vi "LabVIEWArduino1.vi"() -> ()   [LabVIEW 2020]
uses:
  <vilib>/Instr/_visa.llb/VISA Configure Serial Port (Instr).vi
panel:
  out "GO DOWN ECHO 2":string
  out "GO UP ECHO":string
  in  "GO UP":bool
  in  "GO DOWN":bool
  out "MAX SPEED ECHO":string
  out "SLOW SPEED ECHO":string
  in  "MAX SPEED":bool
  in  "SLOWEST SPEED":bool
  out "Waveform Graph":dbl[](graph)
  in  "VISA resource name":refnum<visa-resource-name>="COM3"
  in  "data bits (8)":u16=8 min=5 max=8 step=1
  in  "stop bits (10: 1 bit)":u16(ring)=10 items=["1.0"=10, "1.5"=15, "2.0"=20]
  in  "flow control (0:none)":u16(ring) items=["None", "XON/XOFF", "RTS/CTS", "XON/XOFF & RTS/CTS", "DTR/DSR", "XON/XOFF & DTR/DSR"]
  in  "parity (0:none)":enum16{"None", "Odd", "Even", "Mark", "Space"}(ring)
  out "TempArray":dbl[](array[numeric]) caption="Temperature Array"
  out "CurTemp":dbl caption="Current Temperature\n(Celsius)"
  out "concatenated string":string
  in  "stop":bool
  in  "LabVIEW Stop":bool
  out "LabVIEW Echo":string
  out "Emergency Stop Echo":string
  in  "Emergency Stop!":bool
  out "DECELLERATE ECHO":string
  in  "Decellerate":bool
  in  "Motor Control Duino":refnum<visa-resource-name>
  out "ACCELERATE VALUE CHANGE":string
  in  "Accelerate":bool
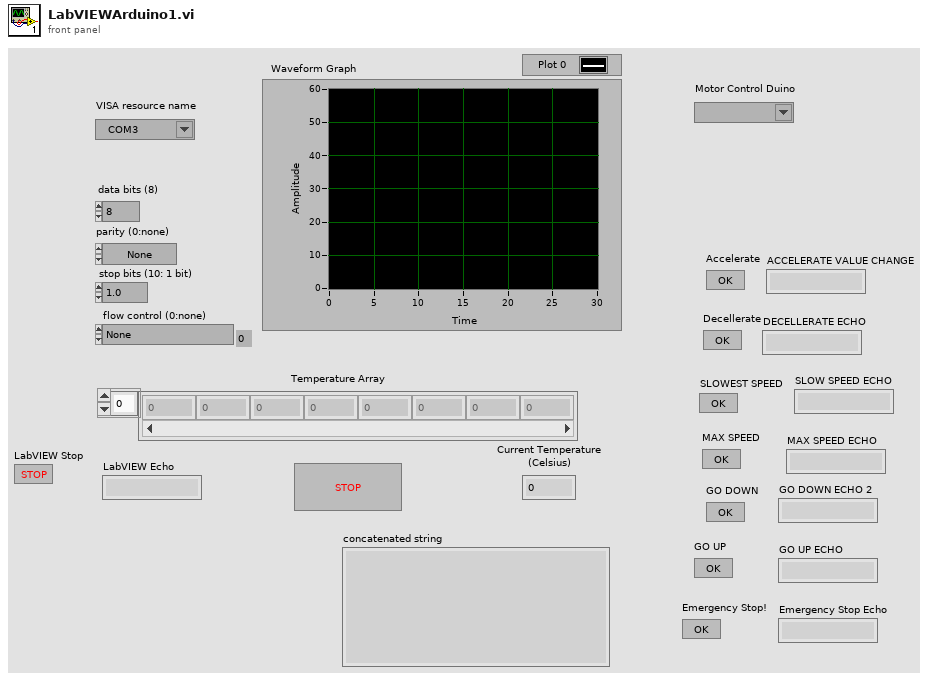
[diagram p1: front panel]
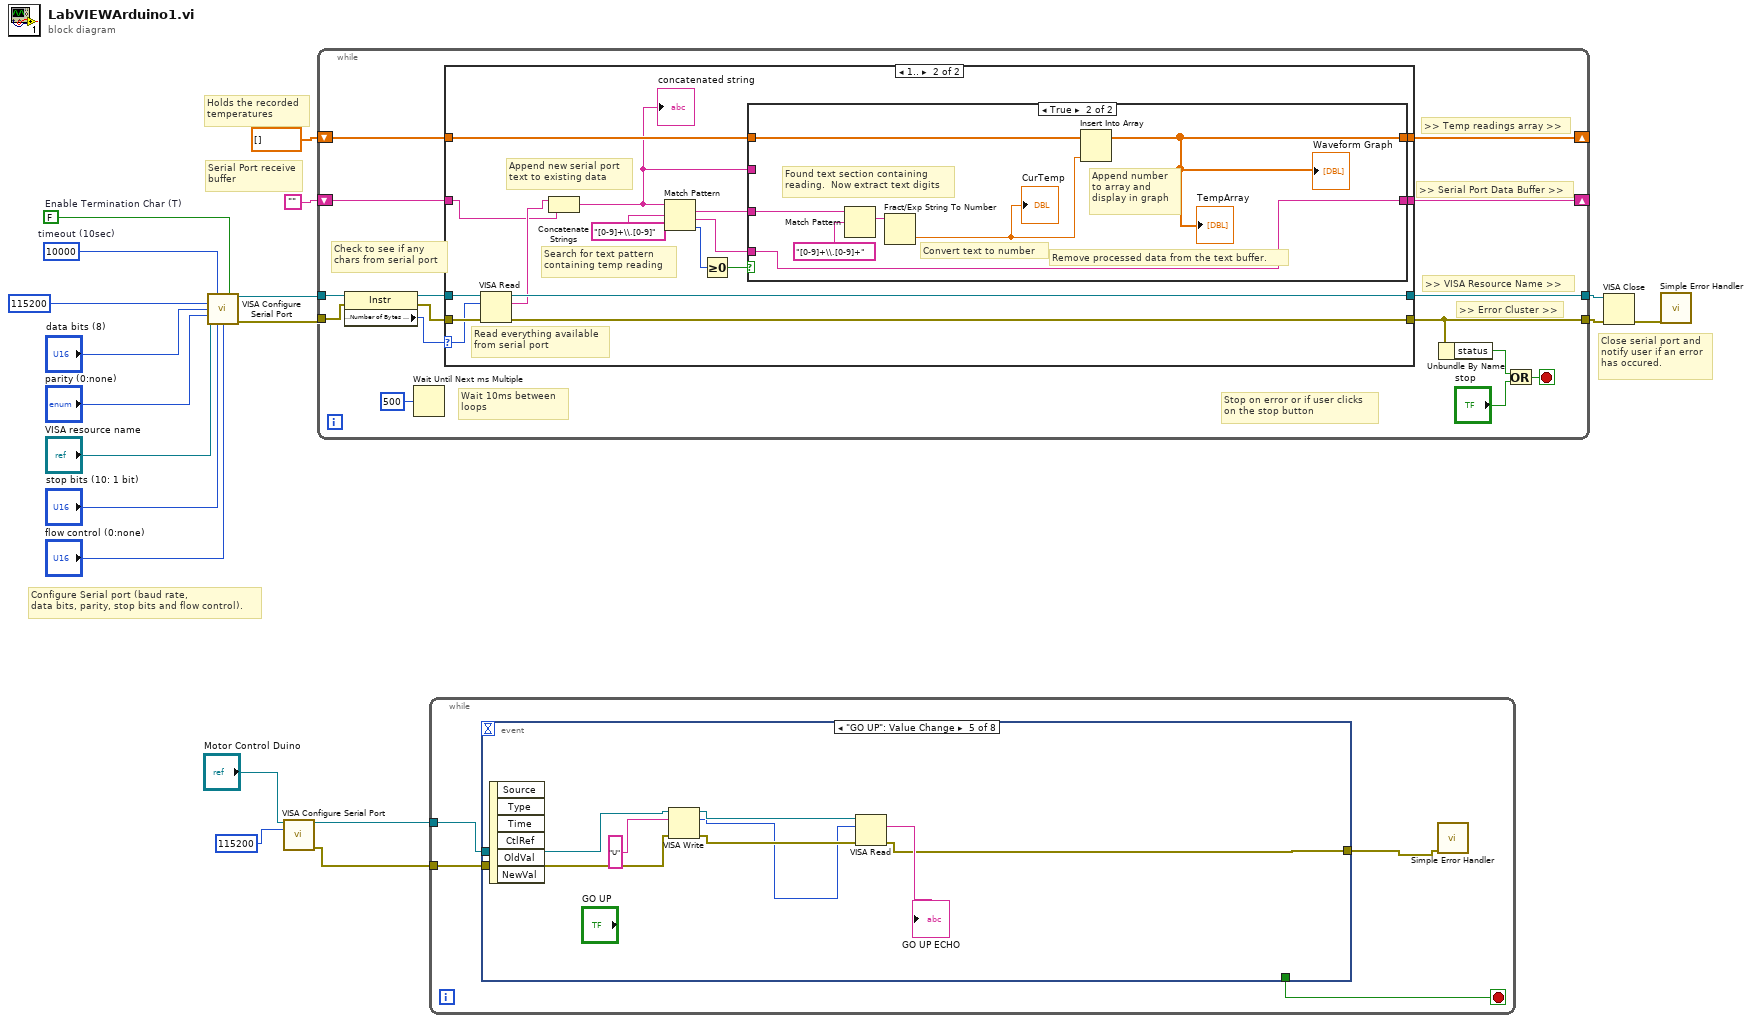
[diagram p0: block diagram]
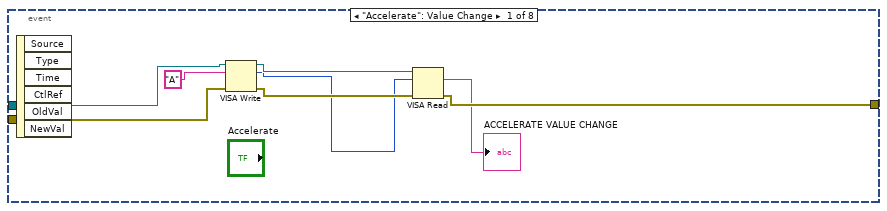
[diagram p4: hidden frame]
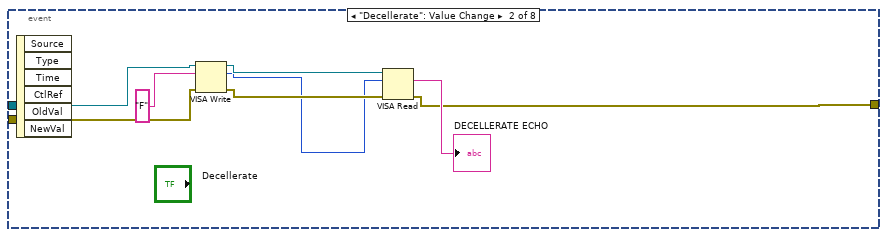
[diagram p5: hidden frame]
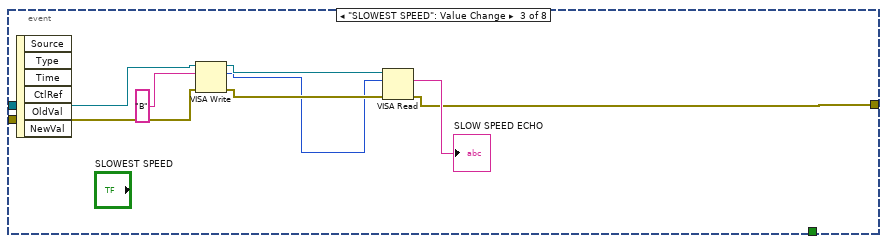
[diagram p6: hidden frame]
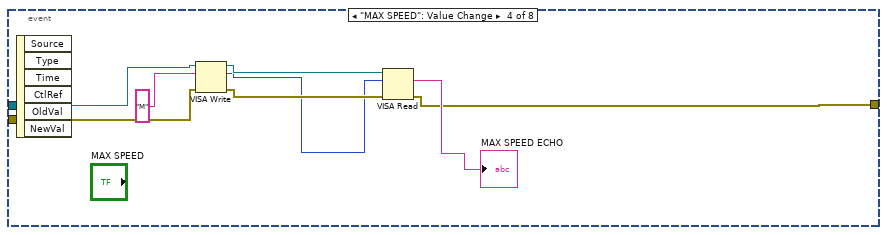
[diagram p7: hidden frame]
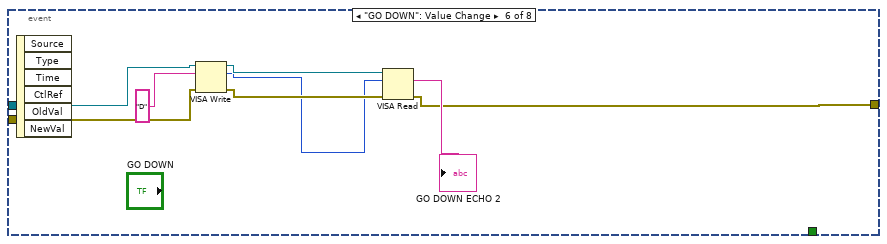
[diagram p8: hidden frame]
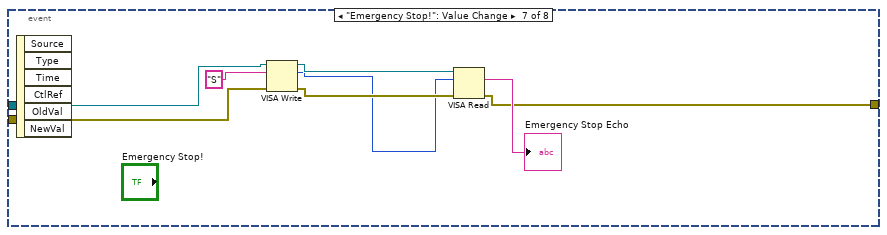
[diagram p9: hidden frame]
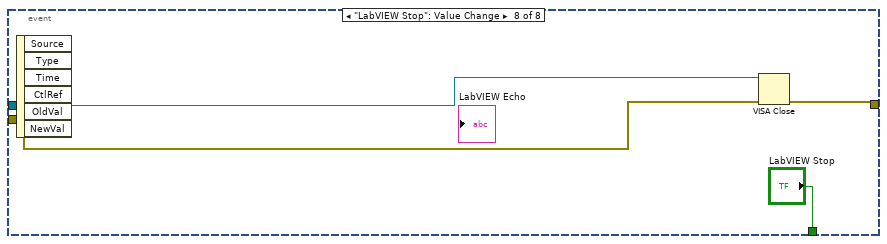
[diagram p10: hidden frame]
diagram:
  w11 = FALSE  # Enable Termination Char (T)
  w12 = u32 10000  # timeout (10sec)
  # "Close serial port and\nnotify user if an error\nhas occured."
  # "Serial Port receive\nbuffer"
  # "Holds the recorded\ntemperatures"
  # "Configure Serial port (baud rate,\ndata bits, parity, stop bits and flow control)."
  n1 = call-poly "VISA Configure Serial Port"("VISA resource name"="VISA resource name", "timeout (10sec)"=w12, "Enable Termination\nChar (T)"=w11, "baud rate (9600)"=u32 115200, "data bits (8)"="data bits (8)", "parity (0:none)"="parity (0:none)", "stop bits (10: 1 bit)"="stop bits (10: 1 bit)", "flow control (0:none)"="flow control (0:none)") -> ("VISA resource name out"=w9:refnum<visa-resource-name>, "error out"=w10:errorcluster)  [unwired: 6 in]
  n2 = call-poly "VISA Configure Serial Port"("VISA resource name"="Motor Control Duino", "baud rate (9600)"=u32 115200) -> ("VISA resource name out"=w19:refnum<visa-resource-name>, "error out"=w18:errorcluster)  [unwired: 12 in]
  n3 = while {
    tunnel: [w26] -> w15
    tunnel: [w34] -> w14
    shift-right: [w20] -> _
    shift-left: "" -> [w28]
    tunnel: w9 -> [w31]
    tunnel: w10 -> [w30]
    shift-right: [w22] -> _
    shift-left: dbl[] [] -> [w21]
    stop <- w25 stop-if-true
    # "Wait 10ms between \nloops"
    # "Stop on error or if user clicks \non the stop button"
    # ">> Error Cluster >>"
    # ">> VISA Resource Name >>"
    # ">> Temp readings array >>"
    # ">> Serial Port Data Buffer >>"
    # "Check to see if any\nchars from serial port"
    n4 = property class="Instr"(reference=w31, error in=w30) -> (reference out=w33:refnum<visa-resource-name>, error out=w32:errorcluster, "Serial Settings:Number of Bytes at Serial Port"=w29:u32)
    n5 = Wait Until Next ms Multiple(millisecond multiple=u32 500) -> ()  [unwired: 1 out]
    n6 = case shown="1.." w29 {
      selector: w29 -> [_ w50]
      tunnel: [w37 w54] -> w26
      tunnel: [w38 w53] -> w34
      tunnel: w33 -> [w38 w52]
      tunnel: w32 -> [w37 w51]
      tunnel: w28 -> [w36 w39]
      tunnel: [w36 w44] -> w20
      tunnel: [w35 w42] -> w22
      tunnel: w21 -> [w35 w43]
      frame 0, Default {
        # "No data in from serial port - Nothing to do."
      }
      frame 1.. {
        # "Search for text pattern\ncontaining temp reading"
        # "Append new serial port\ntext to existing data"
        # "Read everything available\nfrom serial port"
        n7 = VISA Read(VISA resource name=w52, byte count=w50, error in (no error)=w51) -> (VISA resource name out=w53:refnum<visa-resource-name>, read buffer=w40:string, error out=w54:errorcluster)  [unwired: 1 out]
        n8 = Concatenate Strings(w40, w39) -> (w41:string)
        "concatenated string" <- w41
        n9 = Match Pattern(string=w41, regular expression="[0-9]+\\.[0-9]") -> (match substring=w46:string, after substring=w45:string, offset past match=w48:i32)  [unwired: 1 in, 1 out]
        n10 = Greater Or Equal To 0?(x=w48) -> (x >= 0?=w47:bool)
        n11 = case shown="True" w47 {
          tunnel: w46 -> [_ w62]
          tunnel: w45 -> [_ w63]
          tunnel: w41 -> [w56 _]
          tunnel: [w56 w63] -> w44
          tunnel: [w55 w57] -> w42
          tunnel: w43 -> [w55 w60]
          frame False {
            # "Did not find text pattern in the buffer.  Try again in the next loop after new data \nhas been received."
          }
          frame True {
            # "Remove processed data from the text buffer."
            # "Append number\nto array and\ndisplay in graph"
            # "Convert text to number"
            # "Found text section containing \nreading.  Now extract text digits"
            n12 = Match Pattern(string=w62, regular expression="[0-9]+\\.[0-9]+") -> (match substring=w61:string)  [unwired: 1 in, 3 out]
            n13 = Fract/Exp String To Number(string=w61) -> (number=w58:dbl)  [unwired: 3 in, 1 out]
            "CurTemp" <- w58
            n14 = Insert Into Array(array=w60, new element=w58) -> (w57:dbl[])  [unwired: 1 in]
            "TempArray" <- w57
            "Waveform Graph" <- w57
          }
        }
      }
    }
    n15 = Unbundle By Name(w26) -> ("status"=w24:bool)
    n16 = Or(x=w24, y="stop") -> (x .or. y?=w25:bool)
  }
  n17 = while {
    tunnel: w19 -> [w67]
    tunnel: w18 -> [w66]
    stop <- w64 stop-if-true
    n18 = event shown="[4] \"GO UP\": Value Change" {
      selector: _ -> [_ _ _ _ _ _ _ _]
      dyn-events: _ -> [_ _ _ _ _ _ _ _]
      timeout: _ -> [_ _ _ _ _ _ _ _]
      tunnel: [w75 w76 w84 w92 w100 w108 w116 w127] -> w65
      tunnel: w67 -> [w71 w78 w86 w94 w102 w110 w118 w126]
      tunnel: w66 -> [w70 w77 w85 w93 w101 w109 w117 w125]
      tunnel: [_ _ _ _ _ _ _ "LabVIEW Stop"] -> w64
      event "Accelerate": Value Change {
        n19 = event-data() -> ()  [unwired: 1 in, 6 out]
        n20 = VISA Write(VISA resource name=w71, write buffer="A", error in (no error)=w70) -> (VISA resource name out=w73:refnum<visa-resource-name>, return count=w69:u32, error out=w72:errorcluster)
        n21 = VISA Read(VISA resource name=w73, byte count=w69, error in (no error)=w72) -> (read buffer=→"ACCELERATE VALUE CHANGE":string, error out=w75:errorcluster)  [unwired: 2 out]
      }
      event "Decellerate": Value Change {
        n22 = event-data() -> ()  [unwired: 1 in, 6 out]
        n23 = VISA Write(VISA resource name=w78, write buffer="F", error in (no error)=w77) -> (VISA resource name out=w82:refnum<visa-resource-name>, return count=w80:u32, error out=w81:errorcluster)
        n24 = VISA Read(VISA resource name=w82, byte count=w80, error in (no error)=w81) -> (read buffer=→"DECELLERATE ECHO":string, error out=w76:errorcluster)  [unwired: 2 out]
      }
      event "SLOWEST SPEED": Value Change {
        n25 = event-data() -> ()  [unwired: 1 in, 6 out]
        n26 = VISA Write(VISA resource name=w86, write buffer="B", error in (no error)=w85) -> (VISA resource name out=w90:refnum<visa-resource-name>, return count=w88:u32, error out=w89:errorcluster)
        n27 = VISA Read(VISA resource name=w90, byte count=w88, error in (no error)=w89) -> (read buffer=→"SLOW SPEED ECHO":string, error out=w84:errorcluster)  [unwired: 2 out]
      }
      event "MAX SPEED": Value Change {
        n28 = event-data() -> ()  [unwired: 1 in, 6 out]
        n29 = VISA Write(VISA resource name=w94, write buffer="M", error in (no error)=w93) -> (VISA resource name out=w98:refnum<visa-resource-name>, return count=w96:u32, error out=w97:errorcluster)
        n30 = VISA Read(VISA resource name=w98, byte count=w96, error in (no error)=w97) -> (read buffer=→"MAX SPEED ECHO":string, error out=w92:errorcluster)  [unwired: 2 out]
      }
      event "GO UP": Value Change {
        n31 = event-data() -> ()  [unwired: 1 in, 6 out]
        n32 = VISA Write(VISA resource name=w102, write buffer="U", error in (no error)=w101) -> (VISA resource name out=w106:refnum<visa-resource-name>, return count=w104:u32, error out=w105:errorcluster)
        n33 = VISA Read(VISA resource name=w106, byte count=w104, error in (no error)=w105) -> (read buffer=→"GO UP ECHO":string, error out=w100:errorcluster)  [unwired: 2 out]
      }
      event "GO DOWN": Value Change {
        n34 = event-data() -> ()  [unwired: 1 in, 6 out]
        n35 = VISA Write(VISA resource name=w110, write buffer="D", error in (no error)=w109) -> (VISA resource name out=w114:refnum<visa-resource-name>, return count=w112:u32, error out=w113:errorcluster)
        n36 = VISA Read(VISA resource name=w114, byte count=w112, error in (no error)=w113) -> (read buffer=→"GO DOWN ECHO 2":string, error out=w108:errorcluster)  [unwired: 2 out]
      }
      event "Emergency Stop!": Value Change {
        n37 = event-data() -> ()  [unwired: 1 in, 6 out]
        n38 = VISA Write(VISA resource name=w118, write buffer="S", error in (no error)=w117) -> (VISA resource name out=w122:refnum<visa-resource-name>, return count=w120:u32, error out=w121:errorcluster)
        n39 = VISA Read(VISA resource name=w122, byte count=w120, error in (no error)=w121) -> (read buffer=→"Emergency Stop Echo":string, error out=w116:errorcluster)  [unwired: 2 out]
      }
      event "LabVIEW Stop": Value Change {
        n40 = event-data() -> ()  [unwired: 1 in, 6 out]
        n41 = VISA Close(VISA resource name=w126, error in (no error)=w125) -> (error out=w127:errorcluster)
      }
    }
    n42 = call <vilib>:"Simple Error Handler.vi"("error in (no error)"=w65) -> ()  [unwired: 4 in, 5 out]
  }
  n43 = VISA Close(VISA resource name=w14, error in (no error)=w15) -> (error out=w13:errorcluster)
  n44 = call <vilib>:"Simple Error Handler.vi"("error in (no error)"=w13) -> ()  [unwired: 4 in, 5 out]
